vi "niLvFpga_Write32_NI 9146.vi"(0 "session in":u32, 7 "address":u32 format="%.0x", 9 "value":u32 format="%.0x", 11 "error in":errorcluster {"code" format="%.0x"}) -> (4 "session out":u32 caption="reference out", 15 "error out":errorcluster {"code" format="%.0x"})   [LabVIEW 2017]
doc: "Performance related peculiarities:\n\n1. Disable the Call Library Function's \"Generate Wrappers\" feature. This feature is displayed when you add the following labview.ini token, and right click on the Call Library Function node:\nextFuncGenNoWrapperEnabled=True\n\n2. For the Call Library function, enable \"Constant\" for parameters >> session.\n\n3. Remove the error case structure around the Call Library Functions. Chaining the errors between multiple Call Library Functions will suffice."
uses:
  NiFpgaLv.dll
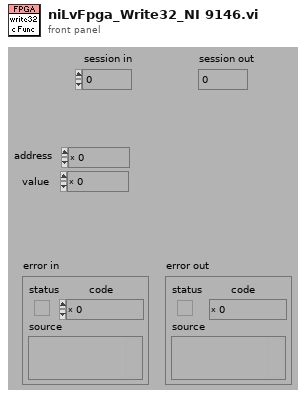
[diagram p1: front panel]
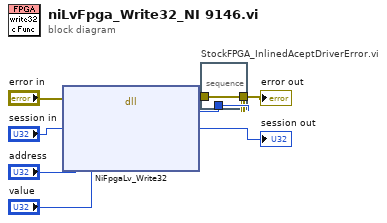
[diagram p0: block diagram]
diagram:
  n1 = dll-call lib="NiFpgaLv.*" fn="NiFpgaLv_Write32" label="niLvFpgaWrite32"(error in="error in", "session"="session in", "address"="address", "value"="value") -> (error out=w5:errorcluster, "status"=w3:i32, "session"=→"session out":u32)  [unwired: 4 in, 1 out]
  n2 = stacked-sequence "StockFPGA_InlinedAceptDriverError.vi" {
    tunnel: w5 -> [w9]
    tunnel: w3 -> [w11]
    tunnel: [w10] -> w4
    frame #0 {
      n3 = case shown="Default" w11 {
        selector: w11 -> [_ w13]
        tunnel: [w12 w15] -> w10
        tunnel: w9 -> [w12 w16]
        frame 0 {
        }
        frame Default {
          n4 = Greater Than 0?(x=w13) -> (x > 0?=w14:bool)
          n5 = call <vilib>:"Error Cluster From Error Code.vi"("is warning? (False)"=w14, "error in (no error)"=w16, "error code (0)"=w13) -> ("error out"=w15:errorcluster)  [unwired: 6 in]
        }
      }
    }
  }
  "error out" <- w4
